vi "Generate_WayPoints_Hopping_CV_Surface.vi"(11 "Input Cluster":T2={"Scan Rate (um/s)"=15.0, "X Start"=15.0, "X End"=15.0, "Y Start"=15.0, "Y End"=15.0, " Z Start"=15.0, "HoppingDistance"=1.0, "V"=15.0, "Z End"=15.0, "Approach Rate Hopping (um/s)"=15.0, "Retrack Rate (um/s)"=15.0, "V 2"=15.0, "Approach Rate (um/s)"=15.0, "V 3"=15.0, "CV Rate / V/s"=15.0, "V 4"=15.0, "V 1"=15.0, "HoldTime1/s"=15.0, "Hold time 2 / s"=15.0, "Hold time 3/ s"=15.0}) -> (0 "output cluster":T1)   [LabVIEW 2023]
uses:
  TypeDefs/WayPointCluster.ctl
  TypeDefsControls/Time.ctl
  User_Vi/Settings.vi
panel:
  in  "WayPointCluster":T1
  out "Y  P":dbl
  out "X  P":dbl
  out "HoppingDistanceX":dbl
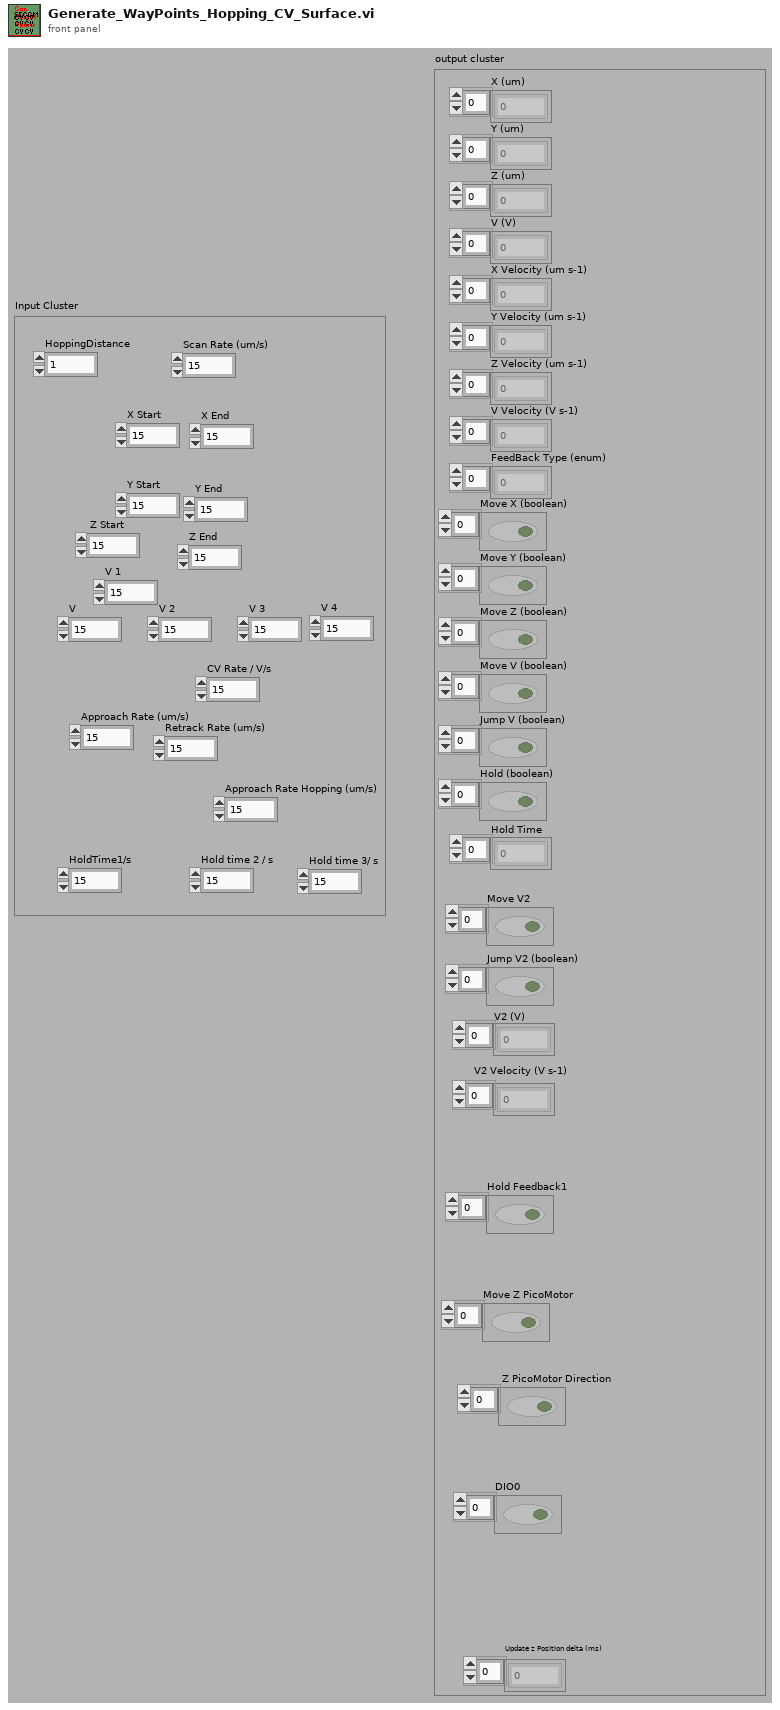
[diagram p1: front panel]
types:
  T1 = typedef "WayPointCluster.ctl" = cluster{"X (um)":dbl[], "Y (um)":dbl[], "Z (um)":dbl[], "V (V)":dbl[], "X Velocity (um s-1)":dbl[], "Y Velocity (um s-1)":dbl[], "Z Velocity (um s-1)":dbl[], "V Velocity (V s-1)":dbl[], "FeedBack Type (enum)":u16[], "Move X (boolean)":bool[], "Move Y (boolean)":bool[], "Move Z (boolean)":bool[], "Move V (boolean)":bool[], "Jump V (boolean)":bool[], "Hold (boolean)":bool[], "Hold Time":u32[], "V2 (V)":dbl[], "Move V2":bool[], "V2 Velocity (V s-1)":dbl[], "Jump V2 (boolean)":bool[], "Update z Position delta (ms)":i16[], "Hold Feedback1":bool[], "Move Z PicoMotor":bool[], " Z PicoMotor Direction":bool[], "DIO0":bool[]}
  T2 = cluster{"Scan Rate (um/s)":dbl, "X Start":dbl, "X End":dbl, "Y Start":dbl, "Y End":dbl, " Z Start":dbl, "HoppingDistance":dbl, "V":dbl, "Z End":dbl, "Approach Rate Hopping (um/s)":dbl, "Retrack Rate (um/s)":dbl, "V 2":dbl, "Approach Rate (um/s)":dbl, "V 3":dbl, "CV Rate / V/s":dbl, "V 4":dbl, "V 1":dbl, "HoldTime1/s":dbl, "Hold time 2 / s":dbl, "Hold time 3/ s":dbl}
  T3 = typedef "Time.ctl" = dbl
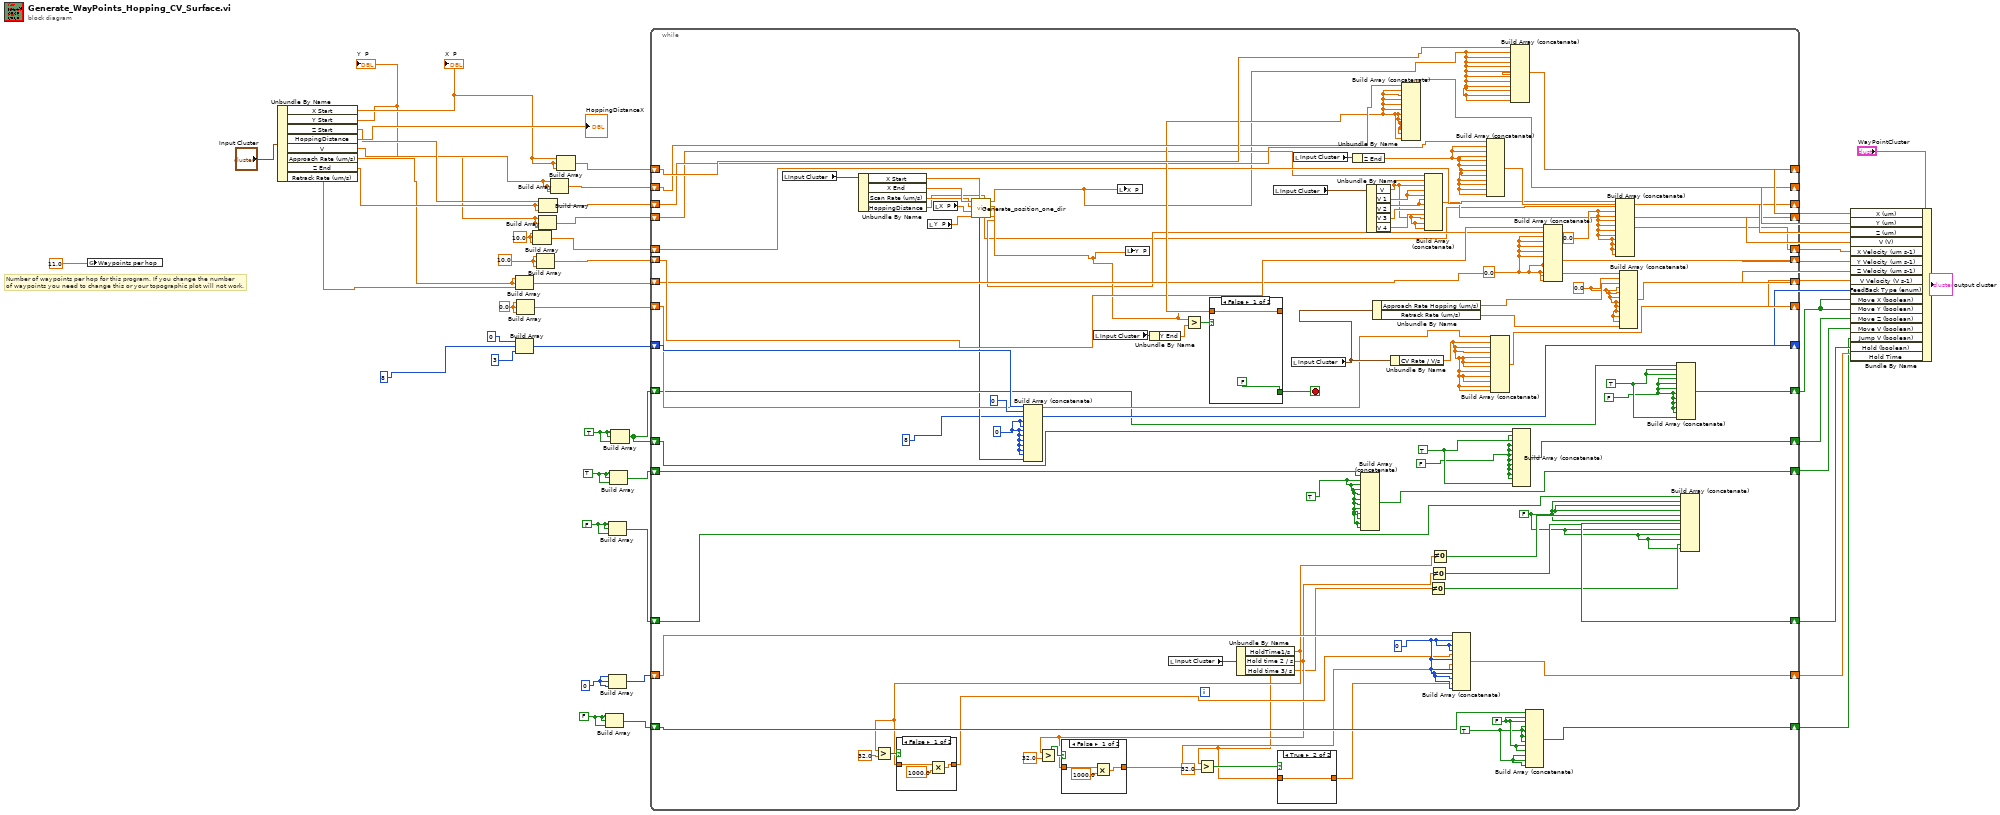
[diagram p0: block diagram]
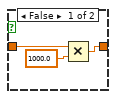
[diagram p2: hidden frame]
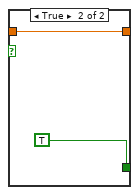
[diagram p5: hidden frame]
diagram:
  w15 = FALSE
  w18 = FALSE
  w17 = u32 0 ("element")
  w16 = TRUE
  w13 = TRUE
  w9 = 10.0 ("element")
  w10 = 10.0 ("element")
  w12 = 0.0 ("element")
  # "Number of waypoints per hop for this program. If you change the number\nof waypoints you need to change this or your topographic plot will not work."
  n1 = global write "Settings.vi" "Waypoints per hop"(11.0) -> ()
  n2 = Unbundle By Name("Input Cluster") -> ("X Start"=w32:dbl, "Y Start"=w31:dbl, "Z Start"=w33:dbl, "HoppingDistance"=→"HoppingDistanceX":dbl, "V"=w29:dbl, "Approach Rate (um/s)"=w11:dbl, "Z End"=w30:dbl, "Retrack Rate (um/s)"=w28:dbl)
  "X  P" <- w32
  "Y  P" <- w31
  n3 = Build Array(w11, w11, w28) -> (w40:dbl[])
  n4 = Build Array(u16 0 ("element"), i16 8, u16 3 ("element")) -> (w36:u16[])
  n5 = Build Array(w12, w12, w12) -> (w38:dbl[])
  n6 = Build Array(w9, w9, w9) -> (w43:dbl[])
  n7 = Build Array(w10, w10, w10) -> (w42:dbl[])
  n8 = Build Array(w29, w29, w29) -> (w45:dbl[])
  n9 = Build Array(w33, w30, w30) -> (w47:dbl[])
  n10 = Build Array(w31, w31, w31) -> (w49:dbl[])
  n11 = Build Array(w32, w32, w32) -> (w51:dbl[])
  n12 = Build Array(w18, w18, w18) -> (w22:bool[])
  n13 = Build Array(w15, w15, w15) -> (w14:bool[])
  n14 = Build Array(w17, w17, w17) -> (w25:u32[])
  n15 = Build Array(w16, w16, w16) -> (w20:bool[])
  n16 = Build Array(w13, w13, w13) -> (w5:bool[])
  n17 = while {
    shift-right: [w129] -> w50
    shift-left: w51 -> [w130]
    shift-right: [w127] -> w48
    shift-left: w49 -> [w128]
    shift-right: [w124] -> w46
    shift-left: w47 -> [w125]
    shift-right: [w116] -> w44
    shift-left: w45 -> [w117]
    shift-right: [w110] -> w26
    shift-left: w43 -> [w122]
    shift-right: [w119] -> w41
    shift-left: w42 -> [w120]
    shift-right: [w108] -> w39
    shift-left: w40 -> [w109]
    shift-right: [w103] -> w37
    shift-left: w38 -> [w104]
    shift-right: [w140] -> w35
    shift-left: w36 -> [w141]
    shift-right: [w100] -> w1
    shift-left: w5 -> [w101]
    shift-right: [w94] -> w24
    shift-left: w14 -> [w95]
    shift-right: [w92] -> w23
    shift-left: w25 -> [w93]
    shift-right: [w56] -> w21
    shift-left: w22 -> [w89]
    shift-right: [w97] -> w2
    shift-left: w20 -> [w98]
    shift-right: [w84] -> w6
    shift-left: w5 -> [w83]
    stop <- w134 stop-if-true
    w86 = FALSE
    w87 = TRUE
    w55 = TRUE
    w121 = 0.0 ("element")
    w96 = TRUE
    w88 = FALSE
    w90 = u32 0 ("element")
    w53 = FALSE
    w85 = FALSE
    w99 = TRUE
    w131 = u16 0 ("element")
    w118 = 0.0 ("element")
    w106 = 0.0 ("element")
    n18 = local read "Input Cluster"() -> (w142:T2)
    n19 = Unbundle By Name(w142) -> ("X Start"=w80:dbl, "X End"=w79:dbl, "Scan Rate (um/s)"=w78:dbl, "HoppingDistance"=w77:dbl)
    n20 = local read "Y  P"() -> (w81:dbl)
    n21 = local read "X  P"() -> (w82:dbl)
    n22 = call "Generate_position_one_dir.vi"("HoppingDistance input"=w77, "X Start input"=w80, "Y P input"=w81, "X P input"=w82, "Scan Rate (um/s) input"=w78, "X end input"=w79) -> ("Y velocity output"=w74:dbl, "Y P output"=w75:dbl, "X P output"=w76:dbl, "X velocity output"=w73:dbl, "Feedback type retraction output"=w72:u64)  [unwired: 1 in]
    n23 = Build Array (concatenate)(w141, u16 0 ("element"), i16 8, w131, w131, w131, w131, w131, w131, w131, w131, w72) -> (w140:u64[])
    n24 = local read "Input Cluster"() -> (w137:T2)
    n25 = local write "X  P"(w76) -> ()
    n26 = local write "Y  P"(w75) -> ()
    n27 = Unbundle By Name(w137) -> ("Y End"=w136:dbl)
    n28 = local read "Input Cluster"() -> (w91:T2)
    n29 = Greater?(x=w75, y=w136) -> (0:w135:bool)
    n30 = case shown="False" w135 {
      tunnel: w75 -> [w156 w158]
      tunnel: [w156 w158] -> w126
      tunnel: [FALSE TRUE] -> w134
      frame False {
      }
      frame True {
      }
    }
    n31 = Unbundle By Name(w91) -> ("HoldTime1/s"=w61:dbl, "Hold time 2 / s"=w59:dbl, "Hold time 3/ s"=w57:dbl)
    n32 = Greater?(x=w61, y=T3 32.0) -> (0:w67:bool)
    n33 = case shown="False" w67 {
      tunnel: w61 -> [w149 w150]
      tunnel: [w148 w150] -> w64
      frame False {
        n34 = Multiply(x=w149, y=1000.0) -> (x*y=w148:dbl)
      }
      frame True {
      }
    }
    n35 = Greater?(x=w59, y=T3 32.0) -> (0:w69:bool)
    n36 = case shown="False" w69 {
      tunnel: w59 -> [w153 w154]
      tunnel: [w152 w154] -> w63
      frame False {
        n37 = Multiply(x=w153, y=1000.0) -> (x*y=w152:dbl)
      }
      frame True {
      }
    }
    n38 = Greater?(x=w57, y=T3 32.0) -> (0:w65:bool)
    n39 = local read "Input Cluster"() -> (w138:T2)
    n40 = case shown="True" w65 {
      tunnel: w57 -> [w145 w146]
      tunnel: [w144 w146] -> w62
      frame False {
        n41 = Multiply(x=w145, y=1000.0) -> (x*y=w144:dbl)
      }
      frame True {
      }
    }
    n42 = local read "Input Cluster"() -> (w132:T2)
    n43 = local read "Input Cluster"() -> (w139:T2)
    n44 = Unbundle By Name(w139) -> ("Z End"=w123:dbl)
    n45 = Build Array (concatenate)(w98, w96, w96, w96, w96, w96, w96, w96, w96, w96, w96, w96) -> (w97:bool[])
    n46 = Unbundle By Name(w138) -> ("V"=w111:dbl, "V 1"=w115:dbl, "V 2"=w114:dbl, "V 3"=w113:dbl, "V 4"=w112:dbl)
    n47 = Unbundle By Name(w132) -> ("Approach Rate Hopping (um/s)"=w107:dbl, "Retrack Rate (um/s)"=w105:dbl)
    n48 = Unbundle By Name(w132) -> ("CV Rate / V/s"=w102:dbl)
    n49 = Build Array (concatenate)(w128, w126, w126, w126, w126, w126, w126, w126, w126, w126, w126, w126) -> (w127:dbl[])
    n50 = Build Array (concatenate)(w117, w111, w111, w115, w115, w114, w114, w113, w112, w111, w111, w111) -> (w116:dbl[])
    n51 = Not Equal To 0?(x=w57) -> (x != 0?=w54:bool)
    n52 = Not Equal To 0?(x=w59) -> (x != 0?=w58:bool)
    n53 = Not Equal To 0?(x=w61) -> (x != 0?=w60:bool)
    n54 = Build Array (concatenate)(w93, w90, w90, w90, w64, w90, w63, w90, w90, w90, w62, w90) -> (w92:dbl[])
    n55 = Build Array (concatenate)(w125, w123, w123, w123, w123, w123, w123, w123, w123, w123, w123, w123) -> (w124:dbl[])
    n56 = Build Array (concatenate)(w104, w102, w102, w102, w102, w102, w102, w102, w102, w102, w102, w102) -> (w103:dbl[])
    n57 = Build Array (concatenate)(w130, w76, w76, w76, w76, w76, w76, w76, w76, w76, w76, w76) -> (w129:dbl[])
    n58 = Build Array (concatenate)(w101, w85, w99, w85, w85, w85, w85, w85, w85, w85, w85, w99) -> (w100:bool[])
    n59 = Build Array (concatenate)(w89, w88, w88, w55, w55, w55, w55, w88, w88, w55, w55, w55) -> (w56:bool[])
    n60 = Build Array (concatenate)(w120, w74, w118, w118, w118, w118, w118, w118, w118, w118, w118, w118) -> (w119:dbl[])
    n61 = Build Array (concatenate)(w122, w73, w121, w121, w121, w121, w121, w121, w121, w121, w121, w121) -> (w110:dbl[])
    n62 = Build Array (concatenate)(w109, w106, w107, w106, w106, w106, w106, w106, w106, w106, w106, w105) -> (w108:dbl[])
    n63 = Build Array (concatenate)(w83, w87, w87, w86, w86, w86, w86, w86, w86, w86, w86, w87) -> (w84:bool[])
    n64 = Build Array (concatenate)(w95, w53, w53, w53, w60, w53, w58, w53, w53, w53, w54, w53) -> (w94:bool[])
  }
  n65 = Bundle By Name(cluster="WayPointCluster", "X (um)"=w50, "Y (um)"=w48, "Z (um)"=w46, "V (V)"=w44, "X Velocity (um s-1)"=w26, "Y Velocity (um s-1)"=w41, "Z Velocity (um s-1)"=w39, "V Velocity (V s-1)"=w37, "FeedBack Type (enum)"=w35, "Move X (boolean)"=w6, "Move Y (boolean)"=w6, "Move Z (boolean)"=w1, "Move V (boolean)"=w2, "Jump V (boolean)"=w21, "Hold (boolean)"=w24, "Hold Time"=w23) -> (→"output cluster":T1)
